vi "On Timeout.vi"(8 "error in (no error)":errorcluster, 11 "App in":refnum<class "App.lvclass">) -> (0 "error out":errorcluster, 3 "App out":refnum<class "App.lvclass">)   [LabVIEW 2020, in "AR Example.lvlib" / "App.lvclass"]
uses:
  App.lvclass
  App.lvclass/App.ctl
  g_ar_toolkit.capture/CameraStream/CameraStream.lvclass/CameraStream.ctl
  <vilib>/Utility/error.llb/Error Cluster From Error Code.vi
  UI/UI.lvclass
  g_ar_toolkit.capture/CameraStream/CameraStream.lvclass
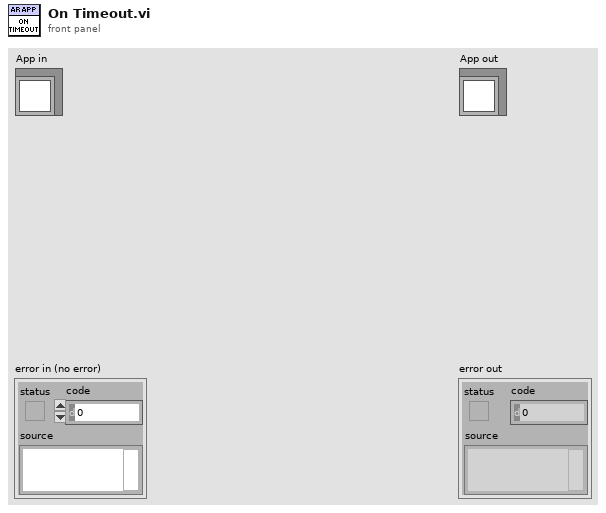
[diagram p1: front panel]
types:
  T1 = typedef "AR Example.lvlib/App.lvclass/Timeout Action.ctl" = enum16{"None", "Capture Preview Image"}
  T2 = typedef "g_ar_toolkit.image.lvlib/Image Draw Offset.ctl" = cluster{"Top":i16, "Left":i16}
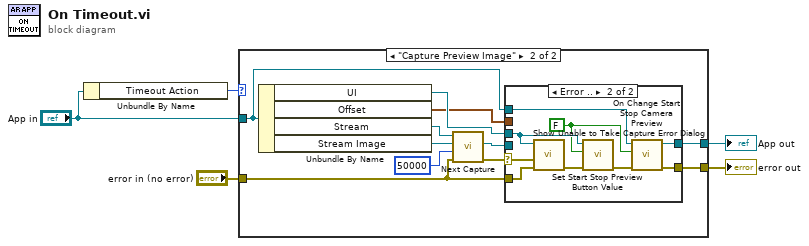
[diagram p0: block diagram]
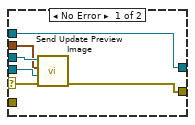
[diagram p3: hidden frame]
diagram:
  n1 = Unbundle By Name("App in") -> ("Timeout Action"=w5:T1)
  n2 = case shown="\"Capture Preview Image\"" w5 {
    tunnel: [w6 w9] -> w4
    tunnel: "App in" -> [w6 w8]
    tunnel: [w7 w13] -> w2
    tunnel: "error in (no error)" -> [w7 w11]
    frame "None" {
    }
    frame "Capture Preview Image" {
      n3 = Unbundle By Name(w8) -> ("UI"=w14:refnum<class "UI.lvclass">, "Offset"=w10:T2, "Stream"=w18:refnum<data-value>, "Stream Image"=w17:refnum<data-value>)
      n4 = call "Next Capture.vi"("error in (no error)"=w11, "timeout (ms)"=u16 50000, "ARGB Image Destination"=w17, "Stream"=w18) -> ("error out"=w15:errorcluster, "ARGB Image (duplicate)"=w12:refnum<data-value>)  [unwired: 5 in, 1 out]
      n5 = case shown="Error .." w15 {
        selector: w15 -> [w23 w30]
        tunnel: w14 -> [w24 w26]
        tunnel: [w22 w31] -> w13
        tunnel: w12 -> [w21 _]
        tunnel: w11 -> [_ w29]
        tunnel: w10 -> [w20 _]
        tunnel: [w19 w32] -> w9
        tunnel: w8 -> [w19 w33]
        frame No Error {
          n6 = call-dynamic "Send Update Preview Image.vi"("error in (no error)"=w23, "Image"=w21, "Draw Offset"=w20, "UI in"=w24) -> ("error out"=w22:errorcluster)  [unwired: 7 in]
        }
        frame Error {
          w25 = FALSE ("Value")
          n7 = call-dynamic "Show Unable to Take Capture Error Dialog.vi"("error in (no error)"=w29, "Stream Start Error"=w30, "UI in"=w26) -> ("error out"=w28:errorcluster)  [unwired: 8 in]
          n8 = call-dynamic "Set Start Stop Preview Button Value.vi"("error in (no error)"=w28, "Values"=w25, "UI in"=w26) -> ("error out"=w27:errorcluster)  [unwired: 8 in]
          n9 = call "On Change Start Stop Camera Preview.vi"("error in (no error)"=w27, "Value"=w25, "App in"=w33) -> ("error out"=w31:errorcluster, "App out"=w32:refnum<class "App.lvclass">)  [unwired: 7 in]
        }
      }
    }
  }
  "error out" <- w2
  "App out" <- w4
